vi "File_combine.vi"() -> ()   [LabVIEW 2019]
uses:
  <vilib>/Utility/file.llb/Read Delimited Spreadsheet (DBL).vi
  <vilib>/Utility/file.llb/Write Delimited Spreadsheet (DBL).vi
panel:
  out "x/y":dbl[](array[numeric])
  out "Array":dbl[](array[numeric])
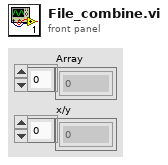
[diagram p1: front panel]
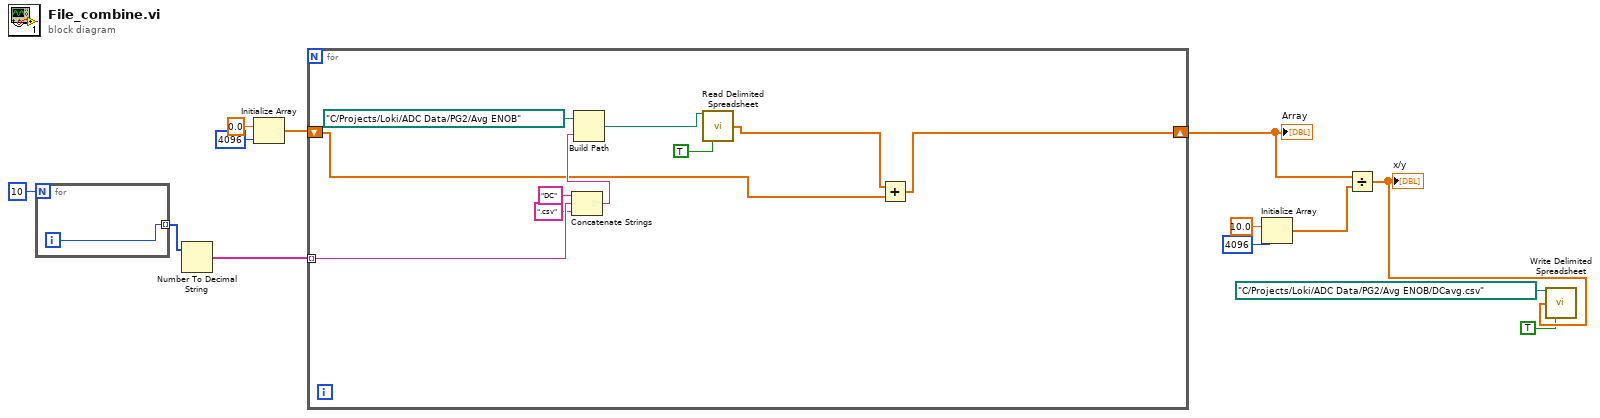
[diagram p0: block diagram]
diagram:
  n1 = for {
    N: 10 -> [_]
    tunnel: [w14] -> w13 mode=indexing
    i -> [w14]
  }
  n2 = Number To Decimal String(number=w13) -> (decimal integer string=w12:string[])  [unwired: 1 in]
  n3 = Initialize Array(0.0 ("element"), 4096 ("dimension size")) -> (w10:dbl[])
  n4 = for {
    tunnel: w12 -> [w21] mode=indexing
    shift-right: [w15] -> w5
    shift-left: w10 -> [w16]
    n5 = Concatenate Strings("DC" ("string"), w21, ".csv" ("string")) -> (w23:string)
    n6 = Build Path(base path=path "C:/Projects/Loki/ADC Data/PG2/Avg ENOB", name or relative path=w23) -> (appended path=w19:path)
    n7 = call-poly <vilib>:"Read Delimited Spreadsheet.vi"("file path (dialog if empty)"=w19, "transpose? (F)"=TRUE) -> ("first row"=w17:dbl[])  [unwired: 8 in, 5 out]
    n8 = Add(x=w17, y=w16) -> (x+y=w15:dbl[])
  }
  "Array" <- w5
  n9 = Initialize Array(10.0 ("element"), 4096 ("dimension size")) -> (w4:dbl[])
  n10 = Divide(x=w5, y=w4) -> (x/y=w2:dbl[])
  "x/y" <- w2
  n11 = call-poly <vilib>:"Write Delimited Spreadsheet.vi"("file path (dialog if empty)"=path "C:/Projects/Loki/ADC Data/PG2/Avg ENOB/DCavg.csv", "1D data"=w2, "transpose? (no:F)"=TRUE) -> ()  [unwired: 11 in, 2 out]
